vi "Loop_HW Servo.vi"   [LabVIEW 2017, in "Gear.lvlib"]
doc: "This example shows how to set and read the angle of a servo.\n\nThis example expects a USB cable connected from your development PC to the Type B USB Jack (next to the power input) on the roboRIO.\n\nThis example requires the Driver Station to be running with Teleoperated Enabled."
uses:
  Gear.lvlib
  Global_CMD to HW.vi
  Globals/Global_HW_Address_Assignments.vi
  Globals/Global_STOP.vi
panel:
  # "Set this input before running."
  # "This can be set while running."
  # "This example requires the Driver Station to be running with Teleoperated Enabled."
  # "PWM cable"
  # "This shows wiring for a HiTEC servo.  The black wire connects to ground (-). The red wire connects to power (V). The white or yellow wire connects to signal (S)."
types:
  T1 = typedef "WPI_ServoDeviceRef.ctl" = cluster{"DeviceStatus":errorcluster, "PWM Channel":T2, "DeadBand":T3}
  T2 = typedef "FPGA_DIOPWMChannel.ctl" = enum8{"PWM 0", "PWM 1", "PWM 2", "PWM 3", "PWM 4", "PWM 5", "PWM 6", "PWM 7", "PWM 8", "PWM 9", "PWM MXP 0", "PWM MXP 1", "PWM MXP 2", "PWM MXP 3", "PWM MXP 4", "PWM MXP 5", "PWM MXP 6", "PWM MXP 7", "PWM MXP 8", "PWM MXP 9", "Invalid"}
  T3 = typedef "WPI_PWMDeadband.ctl" = cluster{"Name":string, "maxPositivePwm":i32, "minPositivePwm":i32, "centerPwm":i32, "maxNegativePwm":i32, "minNegativePwm":i32, "angularRange":u16}
  T4 = typedef "Gear.lvlib/ENUM_Servo Position.ctl" = enum16{"Back", "Forward"}
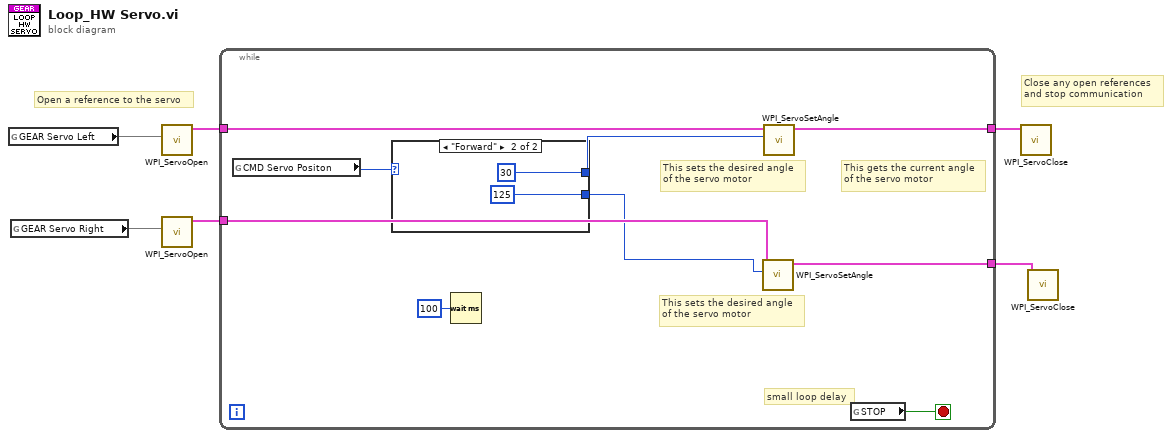
[diagram p0: block diagram]
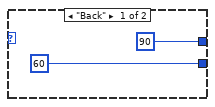
[diagram p2: hidden frame]
diagram:
  # "Close any open references\nand stop communication"
  # "Open a reference to the servo"
  n1 = global read "Global_HW_Address_Assignments.vi" "GEAR Servo Left"() -> (w4)
  n2 = global read "Global_HW_Address_Assignments.vi" "GEAR Servo Right"() -> (w3)
  n3 = call <vilib>:"WPI_ServoOpen.vi"("PWM Channel"=w4) -> ("ServoDeviceRef"=w6:T1)  [unwired: 3 in, 7 out]
  n4 = call <vilib>:"WPI_ServoOpen.vi"("PWM Channel"=w3) -> ("ServoDeviceRef"=w2:T1)  [unwired: 3 in, 7 out]
  n5 = while {
    tunnel: w6 -> [w15]
    tunnel: [w12] -> w5
    tunnel: w2 -> [w11]
    tunnel: [w10] -> w1
    stop <- w14 stop-if-true
    # "This sets the desired angle \nof the servo motor"
    # "small loop delay"
    # "This gets the current angle\nof the servo motor"
    # "This sets the desired angle \nof the servo motor"
    n6 = global read "Global_CMD to HW.vi" "CMD Servo Positon"() -> (w9:T4)
    n7 = case shown="\"Forward\"" w9 {
      tunnel: [60 ("Right") 125 ("Desired Angle")] -> w8
      tunnel: [90 ("Left") 30 ("Desired Angle")] -> w7
      frame "Back" {
      }
      frame "Forward" {
      }
    }
    n8 = Wait (ms)(milliseconds to wait=u32 100) -> ()  [unwired: 1 out]
    n9 = call <vilib>:"WPI_ServoSetAngle.vi"("Angle"=w8, "ServoDeviceRef"=w11) -> ("ServoDeviceRef"=w10:T1)  [unwired: 1 in, 8 out]
    n10 = call <vilib>:"WPI_ServoSetAngle.vi"("Angle"=w7, "ServoDeviceRef"=w15) -> ("ServoDeviceRef"=w12:T1)  [unwired: 1 in, 8 out]
    n11 = global read "Global_STOP.vi" "STOP"() -> (w14:bool)
  }
  n12 = call <vilib>:"WPI_ServoClose.vi"("ServoDeviceRef"=w5) -> ()  [unwired: 1 in, 10 out]
  n13 = call <vilib>:"WPI_ServoClose.vi"("ServoDeviceRef"=w1) -> ()  [unwired: 1 in, 10 out]
